vi "Card counter.vi"(10 "ID":string) -> (2 "# of Cards":i32)   [LabVIEW 2013, in "Universal Power Meter.lvlib" / "WT1600.lvlib" / "WT1600.lvclass"]
uses:
  WT1600.lvclass
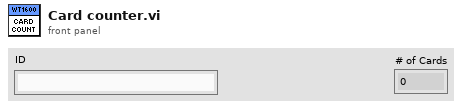
[diagram p1: front panel]
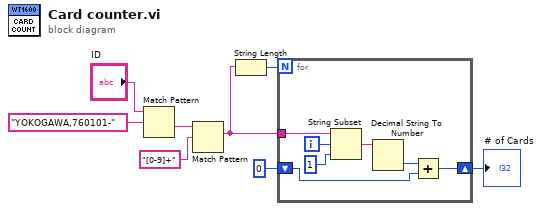
[diagram p0: block diagram]
diagram:
  n1 = Match Pattern(string="ID", regular expression="YOKOGAWA,760101-") -> (after substring=w5:string)  [unwired: 1 in, 3 out]
  n2 = Match Pattern(string=w5, regular expression="[0-9]+") -> (match substring=w3:string)  [unwired: 1 in, 3 out]
  n3 = String Length(string=w3) -> (length=w4:i32)
  n4 = for {
    N: w4 -> [_]
    tunnel: w3 -> [w13]
    shift-right: [w9] -> w1
    shift-left: 0 -> [w10]
    i -> [w14]
    n5 = String Subset(string=w13, offset (0)=w14, length (rest)=1 ("length (rest)")) -> (substring=w12:string)
    n6 = Decimal String To Number(string=w12) -> (number=w11:i32)  [unwired: 2 in, 1 out]
    n7 = Add(x=w11, y=w10) -> (x+y=w9:i32)
  }
  "# of Cards" <- w1
